vi "Set Dashed Tests Ignored.vi"(8 "error in (no error)":errorcluster, 10 "Ingore Dashed?":bool) -> (0 "error out":errorcluster)   [LabVIEW 2020, in "UI Configuration Manager.lvclass"]
uses:
  UI Configuration Manager.lvclass
  Framework/Configuration Manager/Configuration Manager.lvclass
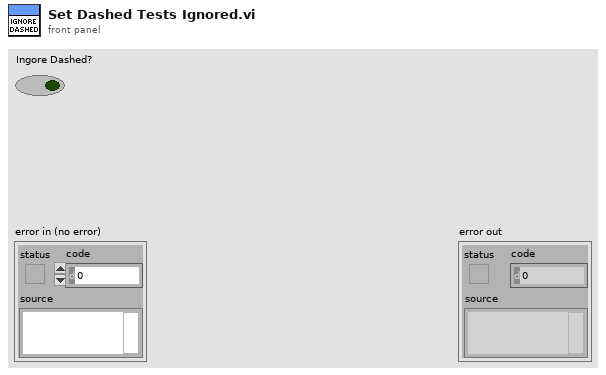
[diagram p1: front panel]
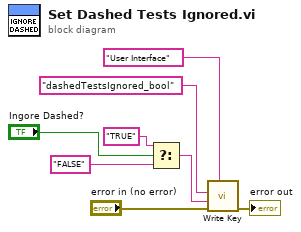
[diagram p0: block diagram]
diagram:
  n1 = Select(t="TRUE" ("key"), s="Ingore Dashed?", f="FALSE") -> (s? t:f=w2:string)
  n2 = call "Write Key.vi"("section"="User Interface", "error in (no error)"="error in (no error)", "value"=w2, "key"="dashedTestsIgnored_bool") -> ("error out"=→"error out":errorcluster)  [unwired: 7 in]
